vi "P3060_DMA写U8数据.vi"(6 "写U8数据":u8[](array[numeric]), 8 "错误输入":errorcluster caption="错误输入（无错误）", 9 "数据长度":u32, 10 "偏移地址":u32, 11 "句柄输入":i32) -> (0 "错误输出":errorcluster, 2 "返回值":i32, 3 "句柄输出":i32)   [LabVIEW 2010]
doc: "发送异步通道数据"
uses:
  dll/P3060.dll
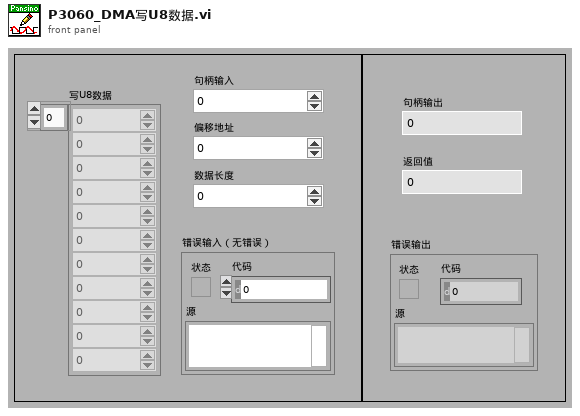
[diagram p1: front panel]
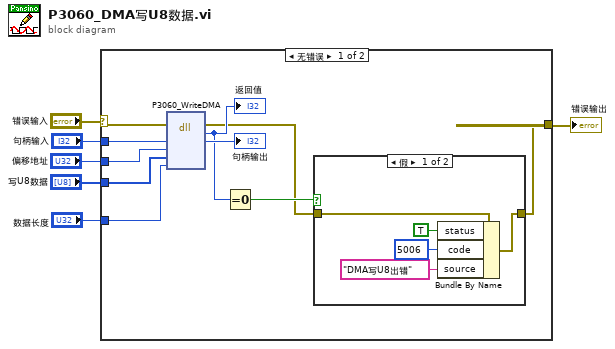
[diagram p0: block diagram]
diagram:
  n1 = case shown="无错误" "错误输入" {
    selector: "错误输入" -> [w16 w23]
    tunnel: [w9 w23] -> w4
    tunnel: "数据长度" -> [w14 _]
    tunnel: "句柄输入" -> [w13 _]
    tunnel: "写U8数据" -> [w8 _]
    tunnel: "偏移地址" -> [w7 _]
    frame No Error {
      n2 = dll-call lib="D:/driver/trunk/Drivers/P3060/P3060API/P3060APILV/Labview/P3060/_SubVI/dll/P3060.dll" fn="P3060_WriteDMA"(error in=w16, "hDev"=w13, "Offset"=w7, "pBuffer"=w8, "lengthToWrite"=w14) -> (error out=w10:errorcluster, "return"=w12:i32, "hDev"=→"句柄输出":i32)  [unwired: 5 in, 1 out]
      "返回值" <- w12
      n3 = Equal To 0?(x=w12) -> (x = 0?=w11:bool)
      n4 = case shown="假" w11 {
        tunnel: [w20 w22] -> w9
        tunnel: w10 -> [w21 w22]
        frame False {
          n5 = Bundle By Name(cluster=w21, "status"=TRUE, "code"=5006, "source"="DMA写U8出错") -> (w20:errorcluster)
        }
        frame True {
        }
      }
    }
    frame Error {
    }
  }
  "错误输出" <- w4
